vi "Post_Build_GetListing.vi"(10 "Files Generated by Build":path[](array[path]), 11 "Runtime Path":path) -> (3 "Files to clear":path[](array[path]))   [LabVIEW 2022 SP3]
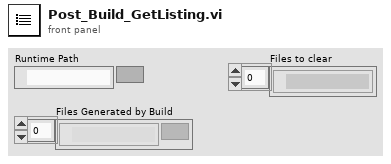
[diagram p1: front panel]
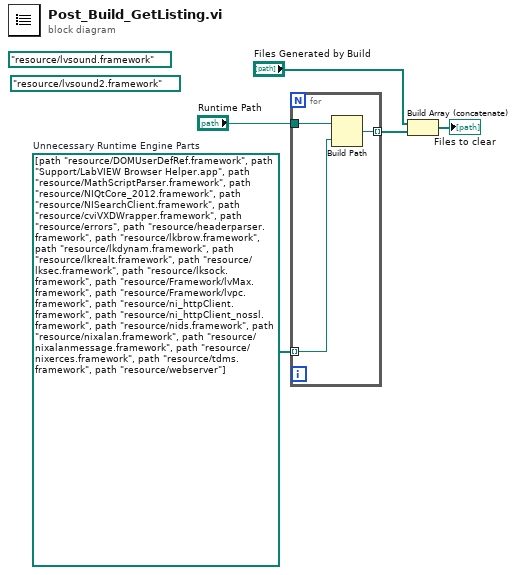
[diagram p0: block diagram]
diagram:
  (unwired) path "resource/lvsound2.framework"
  (unwired) path "resource/lvsound.framework"
  w5 = path[] [path "resource/DOMUserDefRef.framework", path "Support/LabVIEW Browser Helper.app", path "resource/MathScriptParser.framework", path "resource/NIQtCore_2012.framework", path "resource/NISearchClient.framework", path "resource/cviVXDWrapper.framework", path "resource/errors", path "resource/headerparser.framework", path "resource/lkbrow.framework", path "resource/lkdynam.framework", path "resource/lkrealt.framework", path "resource/lksec.framework", path "resource/lksock.framework", path "resource/Framework/lvMax.framework", path "resource/Framework/lvpc.framework", path "resource/ni_httpClient.framework", path "resource/ni_httpClient_nossl.framework", path "resource/nids.framework", path "resource/nixalan.framework", path "resource/nixalanmessage.framework", path "resource/nixerces.framework", path "resource/tdms.framework", path "resource/webserver"]  # Unnecessary Runtime Engine Parts
  n1 = for {
    tunnel: "Runtime Path" -> [w8]
    tunnel: w5 -> [w7] mode=indexing
    tunnel: [w6] -> w2 mode=indexing
    n2 = Build Path(base path=w8, name or relative path=w7) -> (appended path=w6:path)
  }
  n3 = Build Array (concatenate)("Files Generated by Build", w2) -> (→"Files to clear":path[])
